vi "MD5, Convert DBL to MD5.vi"(0 "MD5[0]":dbl=1033964991.0 format="%.1f", 1 "MD5[1]":dbl=3007465432.0 format="%.1f", 2 "MD5[2]":dbl=3077002462.0 format="%.1f", 3 "MD5[3]":dbl=1250560630.0 format="%.1f") -> (4 "int values":u32[](array[numeric]) format="%.0x", 5 "MD5":string)   [LabVIEW 2010]
doc: "This function splits a string of hexadecimal digits (representing an MD5 message-digest) into four unsigned 32-bit integers (8 hexadecimal digits each) then converts the integers to double precision floating point values.\n\nThe inverse of this function is \"MD5, Convert MD5 to DBL.vi\""
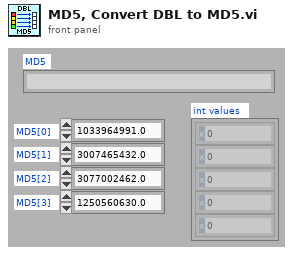
[diagram p1: front panel]
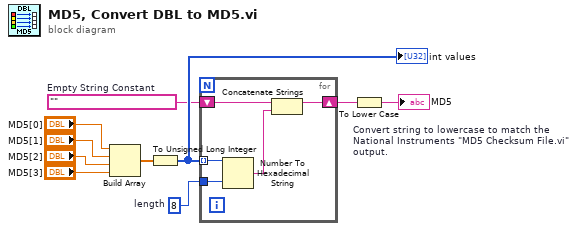
[diagram p0: block diagram]
diagram:
  w3 = 8  # length
  w4 = ""  # Empty String Constant
  n1 = Build Array("MD5[0]", "MD5[1]", "MD5[2]", "MD5[3]") -> (w8:dbl[])
  n2 = To Unsigned Long Integer(number=w8) -> (unsigned 32bit integer=w6:u32[])
  "int values" <- w6
  n3 = for {
    tunnel: w6 -> [w14] mode=indexing
    shift-right: [w12] -> w7
    shift-left: w4 -> [w13]
    tunnel: w3 -> [w11]
    n4 = Number To Hexadecimal String(1:w11, 2:w14) -> (0:w15:string)
    n5 = Concatenate Strings(w13, w15) -> (w12:string)
  }
  n6 = To Lower Case "Convert string to lowercase to match the National Instruments \"MD5 Checksum File.vi\" output."(string=w7) -> (all lower case string=→"MD5":string)
